vi "PDF_Interface_PDF Protokoll EPA1065_LeakCheck.vi"(8 "error in (no error)":errorcluster caption="Fehler (Eingang, kein Fehler)", 10 "TablePictures Refnum In":refnum<vi>[](array[refnum]), 11 "Save PDF File Path":path) -> (0 "error out":errorcluster caption="Fehler (Ausgang)")   [LabVIEW 2020, in "EPA 1065.lvlib" / "Dichtheitstest 1065-345.lvlib"]
uses:
  Dichtheitstest 1065-345.lvlib
  Versa Button.ctl
  VFS Button.ctl
  Sprachverwaltung/FGV Aktion Tabelle zerlegen.ctl
  Aktion Protokolldaten_Leak check.ctl
  Aktion Leak Daten.ctl
  <vilib>/Utility/miscctls.llb/LVRowAndColumnTypeDef.ctl
  <vilib>/Simplicity AI/SAI_PDF_API/Classes/Context/Controls/SAI_PDF_PDF Details.ctl
  PDF_Interface/PDF Interface Helper/PDFContentType.ctl
  PDF_Interface/PDF Interface Helper/PDFTableContentType.ctl
  PDF_Interface/PDF Interface Helper/PDFResults.ctl
  PDF_Interface/PDF Interface Helper/PDFResultPictures.ctl
  PDF_Interface/PDF Interface Helper/PDFCommentPosition.ctl
  PDF_Interface/PDF Interface Helper/PDFPageBreak.ctl
  PDF_Interface/PDF Interface Helper/PDFTablePictures.ctl
  PDF_Interface/PDF Interface Helper/PDFBemerkung.ctl
  <vilib>/Simplicity AI/SAI_PDF_API/Classes/Context/Controls/SAI_PDF_Text Align.ctl
  <vilib>/Simplicity AI/SAI_PDF_API/Classes/Context/Controls/SAI_PDF_Font.ctl
  <vilib>/Simplicity AI/SAI_PDF_API/Classes/Context/Controls/SAI_PDF_Font Encoding.ctl
  PDF_Interface/PDF Protokoll Standard Kopf Optionen.ctl
  Allgemein/allgemeine Sub-VIs.lvlib
  Sprachverwaltung/Sprachverwaltung.lvlib
  PDF_Interface/PDF Interface.lvlib
  <vilib>/Simplicity AI/SAI_PDF_API/Classes/Context/Context.lvclass
  PDF_Interface/PDF Interface Helper/PDF Interface Helper.lvlib
  Linearisierung V2/Protokoll/Protokoll.lvlib
panel:
  in  "VFS button":T1
  in  "FAS button":T2
  out "EPA Konform":string
  out "Inner diameter \nHL to SP":sgl format="%#_5g"
  out "Length HL to SP":sgl format="%#_5g"
  out "Total volume VFS":sgl
  out "Length HL to VFS":sgl format="%#_5g"
  out "Inner diameter  \nHL to VFS":sgl format="%#_5g"
  out "Total volume versa":sgl caption="Total volume Versa"
  out "Heizleitung\nzum\nVFS":bool caption="Heated line\nto\nVFS"
  out "Heizleitung\nzur\nEntnahmestelle":bool caption="Heated Line\nto\nSampling point"
  out "VFS":bool
  out "Tabelle":string[][](table)
  # "Leak Check - EPA § 1065.345"
  # "mm"
  # "mm"
  # "mm³"
  # "mm"
  # "mm"
  # "mm³"
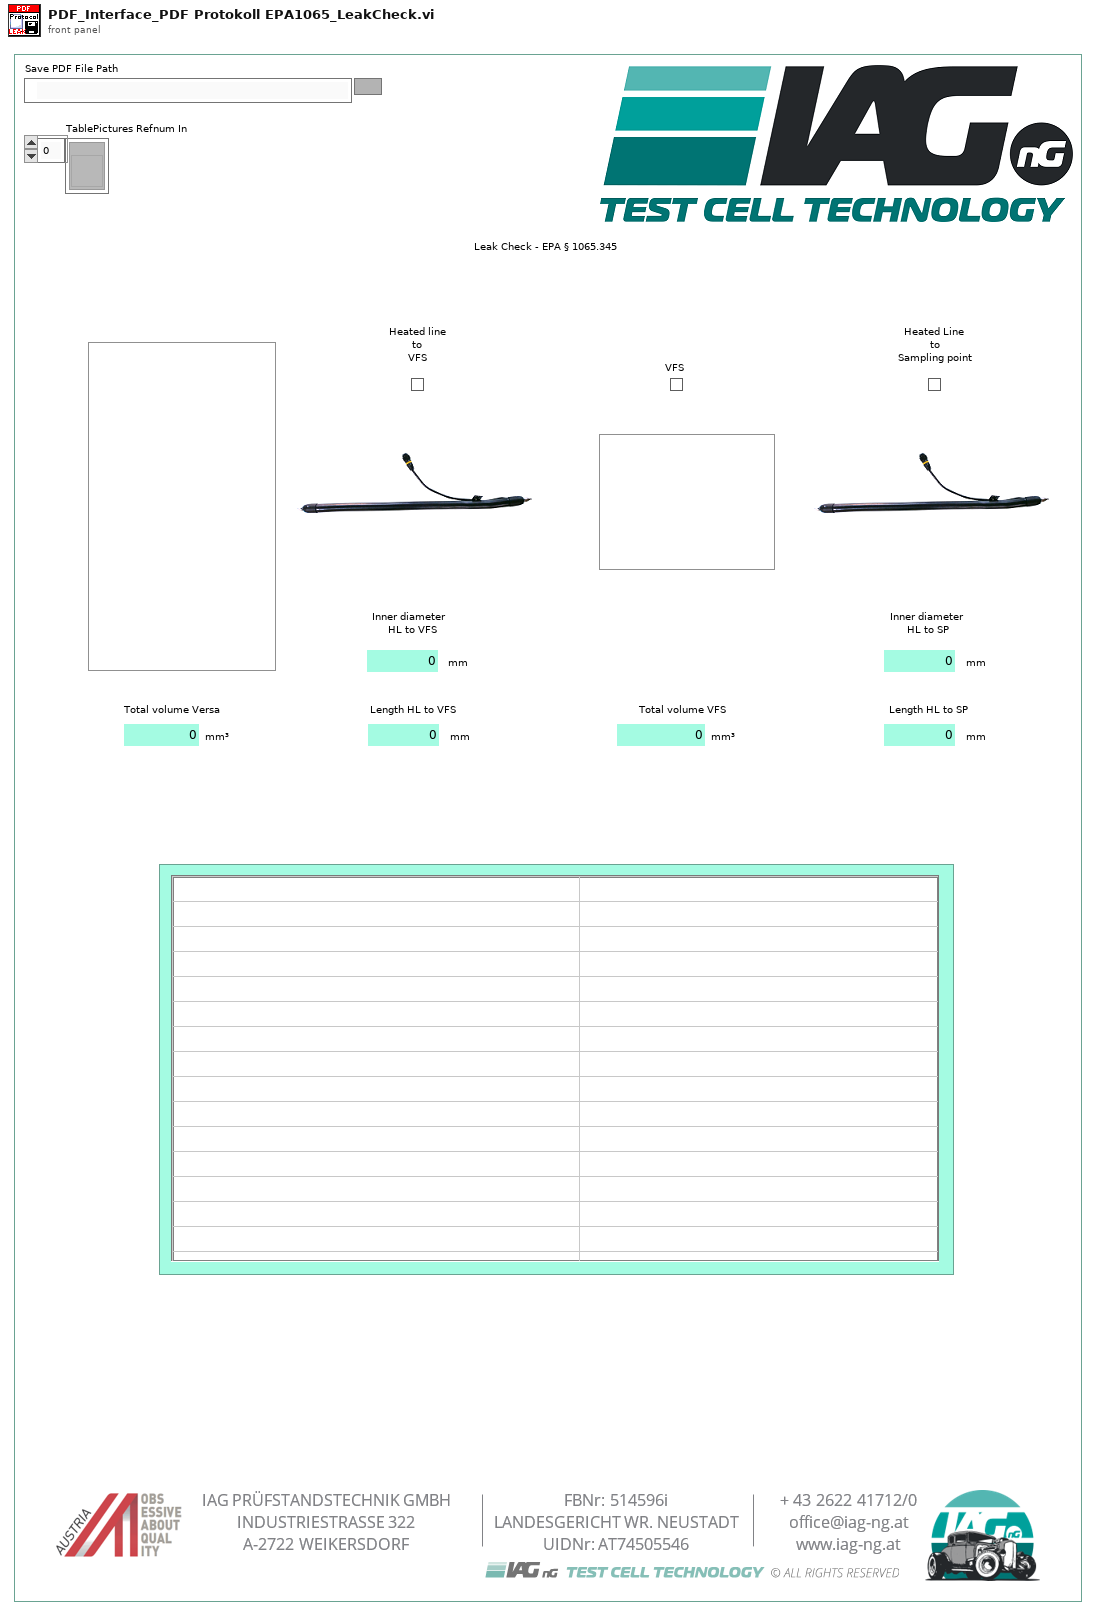
[diagram p1: front panel]
types:
  T1 = typedef "EPA 1065.lvlib/Dichtheitstest 1065-345.lvlib/VFS Button.ctl" = bool
  T2 = typedef "EPA 1065.lvlib/Dichtheitstest 1065-345.lvlib/Versa Button.ctl" = bool
  T3 = typedef "Sprachverwaltung.lvlib/FGV Aktion Tabelle zerlegen.ctl" = enum16{"laden", "vereinzeln", "speichern"}
  T4 = typedef "LVRowAndColumnTypeDef.ctl" = cluster{"Row":i32, "Column":i32}
  T5 = typedef "EPA 1065.lvlib/Dichtheitstest 1065-345.lvlib/Aktion Leak Daten.ctl" = enum16{"lesen", "laden", "speichern", "Volumen", "berechnen", "Leak check aktiv", "Leak Zustand", "Pfad", "Pfad speichern"}
  T6 = typedef "EPA 1065.lvlib/Dichtheitstest 1065-345.lvlib/Aktion Protokolldaten_Leak check.ctl" = enum16{"lesen", "Zeitstempel", "Bearbeiter", "Daten", "Auswertung", "löschen"}
  T7 = typedef "PDF Interface.lvlib/PDF Protokoll Standard Kopf Optionen.ctl" = cluster{"Analysator":bool, "FT-IR Rezept":bool, "Gasteiler":bool, "Gas Komponente":bool, "Gas Flasche":bool, "LIN Protokoll":bool, "Operator":bool}
  T8 = typedef "PDF Interface.lvlib/PDF Interface Helper.lvlib/PDFTablePictures.ctl" = cluster{"Ctl Refnum In":refnum<vi>[], "RowOrColumn":enum16{"Row", "Column"}, "IndexToInsert":u16, "Image Scale (%)":sgl[], "Autoscale? (T)":bool[], "Horizontal Align":i32}
  T9 = typedef "PDF Interface.lvlib/PDF Interface Helper.lvlib/PDFPageBreak.ctl" = enum16{"none", "before", "after", "after comment"}
  T10 = typedef "PDF Interface.lvlib/PDF Interface Helper.lvlib/PDFCommentPosition.ctl" = enum16{"before", "after"}
  T11 = typedef "PDF Interface.lvlib/PDF Interface Helper.lvlib/PDFContentType.ctl" = cluster{"Titel":string, "Header Table":string[][], "Table Array":T12[], "Bemerkungen":T15[]}
  T12 = typedef "PDF Interface.lvlib/PDF Interface Helper.lvlib/PDFTableContentType.ctl" = cluster{"TableHeader":string[], "Table":string[][], "Relative Column Widths (%)":sgl[], "Results":T13, "PositionBemerkung":T10, "PageBreak":T9, "TablePictures":T8, "Horizontal Align":i32}
  T13 = typedef "PDF Interface.lvlib/PDF Interface Helper.lvlib/PDFResults.ctl" = cluster{"Results":cluster{"Result Text":string, "Result":bool}[], "ResultPictures":T14, "use Pictures":bool, "Image Scale (%)":sgl, "Autoscale? (T)":bool, "Horizontal Align":i32, "Position":i32}
  T14 = typedef "PDF Interface.lvlib/PDF Interface Helper.lvlib/PDFResultPictures.ctl" = cluster{"Yes Ctl Refnum":refnum<vi>, "No Ctl Refnum":refnum<vi>}
  T15 = typedef "PDF Interface.lvlib/PDF Interface Helper.lvlib/PDFBemerkung.ctl" = cluster{"Bemerkung Text":string, "Align (Left)":T16, "Add Line Feeds (F:No)":bool, "Font":T17}
  T16 = typedef "SAI_PDF_Toolkit.lvlib/Context.lvclass/SAI_PDF_Text Align.ctl" = i32
  T17 = typedef "SAI_PDF_Toolkit.lvlib/Context.lvclass/SAI_PDF_Font.ctl" = cluster{"Font":string, "Size":i32, "Colour":u32, "Bold":bool, "Italic":bool, "Underline":bool, "Strikethrough":bool, "Font Encoding":T18}
  T18 = typedef "SAI_PDF_Toolkit.lvlib/Context.lvclass/SAI_PDF_Font Encoding.ctl" = enum16{"Cp1252, WinANSI", "IdentityH", "IdentityV", "Cp1250", "Cp1257", "MacRoman"}
  T19 = typedef "SAI_PDF_Toolkit.lvlib/Context.lvclass/SAI_PDF_PDF Details.ctl" = cluster{"Title":string, "Subject":string, "Keywords":string, "Author":string, "Creator":string}
  T20 = cluster{"Header Footer Text Cluster":cluster{"Header Text":string, "Footer Text":string, "Time":string, "Page Number":string}, "PDF Details":T19}
  T21 = typedef "EPA 1065.lvlib/Dichtheitstest 1065-345.lvlib/Gesamtvolumen.ctl" = cluster{"FAS":sgl, "d von HL zu VFS":sgl, "l von HL zu VFS":sgl, "VFS":sgl, "d von HL zu SP":sgl, "l von HL zu SP":sgl, "Heizleitung zum VFS":bool, "VFS a":bool, "Heizleitung zur Entnahmestelle":bool, "Gesamtes Volumen":sgl, "LeakValve":u16, "Einheit":enum16{"mol/s", "mbar"}}
  T22 = typedef "EPA 1065.lvlib/Dichtheitstest 1065-345.lvlib/Leak Protokoll Einstellungen.ctl" = cluster{"Bearbeiter:":string, "Pfad:":path, "Textname:":string, "Analysator":T23}
  T23 = typedef "System Einstellungen V2.lvlib/Analysatoren.ctl" = string
  T24 = cluster{"Header Size":i32, "Column Ratio left":sgl[]}
  T25 = typedef "String - Ausgabefeld.ctl" = string
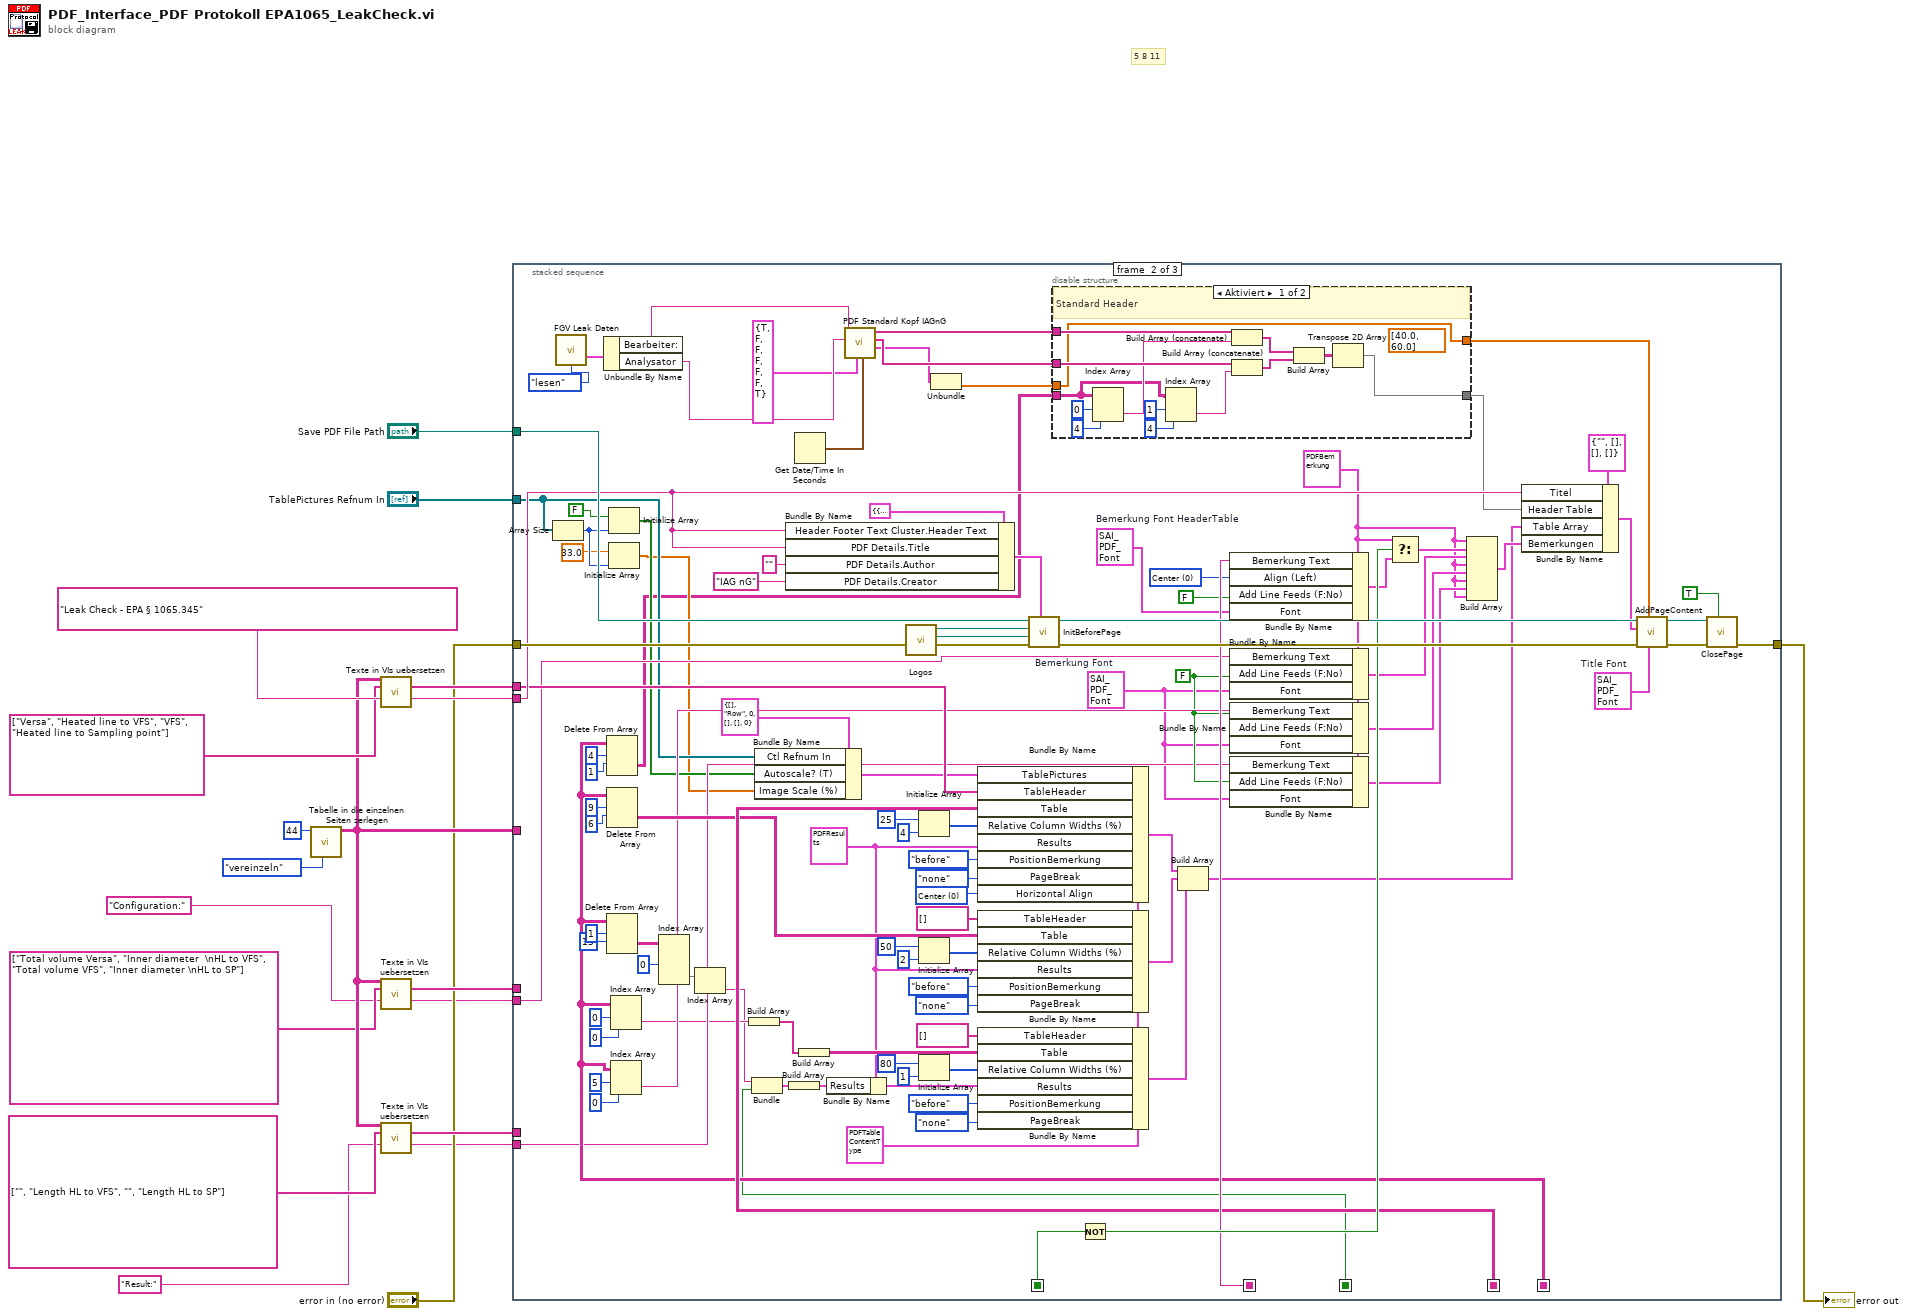
[diagram p0: block diagram]
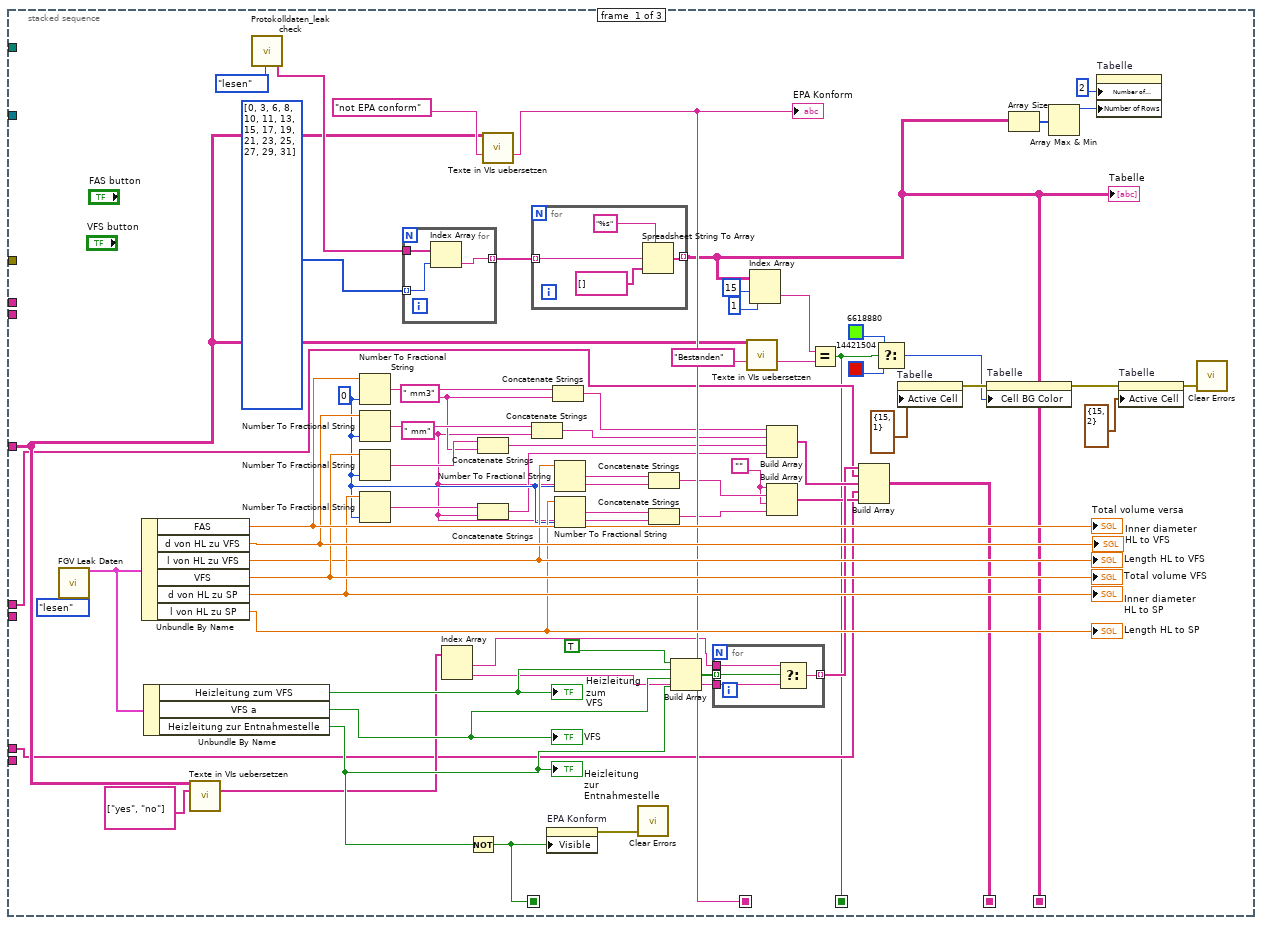
[diagram p2: hidden frame]
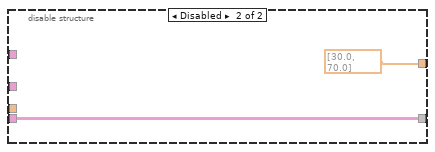
[diagram p3: hidden frame]
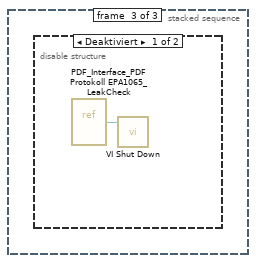
[diagram p4: hidden frame]
diagram:
  # "5 8 11"
  n1 = call "Tabelle in die einzelnen Seiten zerlegen.vi"("Aktion"=FGV_Aktion_Tabelle_zerlegen."vereinzeln", "Index (Seite)"=44) -> ("Sprachliste"=w15:string[][])  [unwired: 7 in, 2 out]
  n2 = call "Texte in VIs uebersetzen.vi"("Sprachliste"=w15, "String-Array zum Übersetzen"=string[] ["Versa", "Heated line to VFS", "VFS", "Heated line to Sampling point"], "String zum Übersetzen"="Leak Check - EPA § 1065.345") -> ("String-Array zum Übersetzen"=w10:string[], "String zum Übersetzen"=w11:string)  [unwired: 8 in, 3 out]
  n3 = call "Texte in VIs uebersetzen.vi"("Sprachliste"=w15, "String-Array zum Übersetzen"=string[] ["Total volume Versa", "Inner diameter  \nHL to VFS", "Total volume VFS", "Inner diameter \nHL to SP"], "String zum Übersetzen"="Configuration:") -> ("String-Array zum Übersetzen"=w12:string[], "String zum Übersetzen"=w4:string)  [unwired: 8 in, 3 out]
  n4 = call "Texte in VIs uebersetzen.vi"("Sprachliste"=w15, "String-Array zum Übersetzen"=string[] ["", "Length HL to VFS", "", "Length HL to SP"], "String zum Übersetzen"="Result:") -> ("String-Array zum Übersetzen"=w9:string[], "String zum Übersetzen"=w2:string)  [unwired: 8 in, 3 out]
  n5 = stacked-sequence {
    seq-local: [w47 _ _] -> [_ w167 _]
    seq-local: [w41 _ _] -> [_ w183 _]
    seq-local: [w40 _ _] -> [_ w145 _]
    seq-local: [w39 _ _] -> [_ w185 _]
    seq-local: [w22 _ _] -> [_ w140 _]
    tunnel: w15 -> [w38 _ _]
    tunnel: w12 -> [w25 _ _]
    tunnel: w11 -> [_ w180 _]
    tunnel: w10 -> [_ w169 _]
    tunnel: w9 -> [w23 _ _]
    tunnel: "Save PDF File Path" -> [_ w189 _]
    tunnel: "error in (no error)" -> [_ w188 _]
    tunnel: [_ w187 _] -> w6
    tunnel: w4 -> [_ w132 _]
    tunnel: w2 -> [_ w129 _]
    tunnel: "TablePictures Refnum In" -> [_ w125 _]
    frame #0 {
      w27 = " mm" ("String")
      w30 = " mm3" ("String")
      w20 = ""
      w48 = i16 0 ("Genauigkeit (6)")
      n6 = call "FGV Leak Daten.vi"("Aktion"=Aktion_Leak_Daten."lesen") -> ("Gesamtvolumen"=w79:T21)  [unwired: 10 in, 4 out]
      n7 = Unbundle By Name(w79) -> ("FAS"=w60:sgl, "d von HL zu VFS"=w58:sgl, "l von HL zu VFS"=w52:sgl, "VFS"=w56:sgl, "d von HL zu SP"=w53:sgl, "l von HL zu SP"=w50:sgl)
      "Total volume versa" <- w60
      "Inner diameter  \nHL to VFS" <- w58
      "Length HL to VFS" <- w52
      "Total volume VFS" <- w56
      "Length HL to SP" <- w50
      "Inner diameter \nHL to SP" <- w53
      n8 = Unbundle By Name(w79) -> ("Heizleitung zum VFS"=w45:bool, "VFS a"=w44:bool, "Heizleitung zur Entnahmestelle"=w43:bool)
      "VFS" <- w44
      "Heizleitung\nzur\nEntnahmestelle" <- w43
      "Heizleitung\nzum\nVFS" <- w45
      n9 = call "Texte in VIs uebersetzen.vi"("Sprachliste"=w38, "String-Array zum Übersetzen"=string[] ["yes", "no"] ("Element")) -> ("String-Array zum Übersetzen"=w36:string[])  [unwired: 9 in, 4 out]
      n10 = call "Protokolldaten_leak check.vi"("Aktion"=Aktion_Protokolldaten_Leak_check."lesen") -> ("Auswertung"=w81:string[])  [unwired: 23 in, 3 out]
      n11 = Number To Fractional String(number=w60, precision (6)=w48) -> (F-format string=w59:string)  [unwired: 2 in]
      n12 = Number To Fractional String(number=w58, precision (6)=w48) -> (F-format string=w57:string)  [unwired: 2 in]
      n13 = Number To Fractional String(number=w56, precision (6)=w48) -> (F-format string=w55:string)  [unwired: 2 in]
      n14 = Number To Fractional String(number=w53, precision (6)=w48) -> (F-format string=w54:string)  [unwired: 2 in]
      n15 = for {
        tunnel: w81 -> [w96]
        tunnel: i32[] [0, 3, 6, 8, 10, 11, 13, 15, 17, 19, 21, 23, 25, 27, 29, 31] -> [w95] mode=indexing
        tunnel: [w94] -> w66 mode=indexing
        n16 = Index Array(array=w96, index=w95) -> (element=w94:string)
      }
      n17 = Index Array(array=w36) -> (element #1=w35:string, element #2=w34:string)  [unwired: 2 in]
      n18 = Not(x=w43) -> (.not. x?=w39:bool)
      n19 = Concatenate Strings(w55, w30) -> (w31:string)
      n20 = Concatenate Strings(w54, w27) -> (w29:string)
      n21 = call "Texte in VIs uebersetzen.vi"("Sprachliste"=w38, "String zum Übersetzen"="not EPA conform" ("EPA Konform")) -> ("String zum Übersetzen"=w41:string)  [unwired: 9 in, 4 out]
      "EPA Konform" <- w41
      n22 = for {
        tunnel: [w92] -> w40 mode=indexing
        tunnel: w66 -> [w90] mode=indexing
        n23 = Spreadsheet String To Array(format string="%s" ("Format-String"), spreadsheet string=w90, array type (2D Dbl)=string[] []) -> (array=w92:string[])  [unwired: 1 in]
      }
      "Tabelle" <- w40
      n24 = Concatenate Strings(w57, w27) -> (w32:string)
      n25 = property on="EPA Konform" class="Str"("Visible"=w39) -> (error out=w63:errorcluster)  [unwired: 2 in, 1 out]
      n26 = Concatenate Strings(w59, w30) -> (w33:string)
      n27 = Number To Fractional String(number=w52, precision (6)=w48) -> (F-format string=w51:string)  [unwired: 2 in]
      n28 = Number To Fractional String(number=w50, precision (6)=w48) -> (F-format string=w49:string)  [unwired: 2 in]
      n29 = call <vilib>:"Clear Errors.vi"("error in (no error)"=w63) -> ()  [unwired: 5 in, 2 out]
      n30 = Concatenate Strings(w51, w27) -> (w28:string)
      n31 = Concatenate Strings(w49, w27) -> (w21:string)
      n32 = Build Array(TRUE, w45, w44, w43) -> (w42:bool[])
      n33 = for {
        tunnel: w42 -> [w89] mode=indexing
        tunnel: [w88] -> w26 mode=indexing
        tunnel: w35 -> [w87]
        tunnel: w34 -> [w86]
        n34 = Select(t=w87, s=w89, f=w86) -> (s? t:f=w88:string)
      }
      n35 = call "Texte in VIs uebersetzen.vi"("Sprachliste"=w38, "String zum Übersetzen"="Bestanden" ("Element")) -> ("String zum Übersetzen"=w76:string)  [unwired: 9 in, 4 out]
      n36 = Index Array(array=w40, index (row)=15 ("Index (Zeile)"), index (col)=1 ("Deaktivierter Index (Spalte)")) -> (element=w74:string)
      n37 = Build Array(w33, w32, w31, w29) -> (w61:string[])
      n38 = Build Array(w20, w28, w20, w21) -> (w24:string[])
      n39 = Equal?(x=w74, y=w76) -> (x = y?=w22:bool)
      n40 = Build Array(w26, w25, w61, w23, w24) -> (w47:string[][])
      n41 = Select(t=u32 6618880, s=w22, f=u32 14421504) -> (s? t:f=w71:u32)
      n42 = property on="Tabelle" class="Tbl (strikt)"("Active Cell"=T4 {"Row"=15, "Column"=1} ("Aktive Zelle:Aktive Zelle")) -> (error out=w72:errorcluster)  [unwired: 2 in, 1 out]
      n43 = property on="Tabelle" class="Tbl (strikt)"(error in=w72, "Cell BG Color"=w71) -> (error out=w70:errorcluster)  [unwired: 1 in, 1 out]
      n44 = Array Size(array=w40) -> (size(s)=w84:i32[])
      n45 = Array Max & Min(array=w84) -> (max value=w83:i32)  [unwired: 3 out]
      n46 = property on="Tabelle" class="Tbl (strikt)"("Number of Columns"=u32 2 ("Spaltenanzahl"), "Number of Rows"=w83) -> ()  [unwired: 2 in, 2 out]
      n47 = property on="Tabelle" class="Tbl (strikt)"(error in=w70, "Active Cell"=T4 {"Row"=15, "Column"=2} ("Aktive Zelle:Aktive Zelle")) -> (error out=w68:errorcluster)  [unwired: 1 in, 1 out]
      n48 = call <vilib>:"Clear Errors.vi"("error in (no error)"=w68) -> ()  [unwired: 5 in, 2 out]
    }
    frame #1 {
      w112 = T15 {"Bemerkung Text"="", "Align (Left)"=0, "Add Line Feeds (F:No)"=FALSE, "Font"={"Font"="Arial", "Size"=10, "Colour"=0, "Bold"=FALSE, "Italic"=FALSE, "Underline"=FALSE, "Strikethrough"=FALSE, "Font Encoding"=enum."Cp1252, WinANSI"}} ("Bemerkung")
      w114 = T13 {"Results"=[], "ResultPictures"={"Yes Ctl Refnum"=refnum, "No Ctl Refnum"=refnum}, "use Pictures"=FALSE, "Image Scale (%)"=100.0, "Autoscale? (T)"=TRUE, "Horizontal Align"=3, "Position"=0} ("Results")
      w116 = T12 {"TableHeader"=[], "Table"=[], "Relative Column Widths (%)"=[], "Results"={"Results"=[], "ResultPictures"={"Yes Ctl Refnum"=refnum, "No Ctl Refnum"=refnum}, "use Pictures"=FALSE, "Image Scale (%)"=0.0, "Autoscale? (T)"=FALSE, "Horizontal Align"=0, "Position"=0}, "PositionBemerkung"=enum."before", "PageBreak"=enum."none", "TablePictures"={"Ctl Refnum In"=[], "RowOrColumn"=enum."Row", "IndexToInsert"=0, "Image Scale (%)"=[], "Autoscale? (T)"=[], "Horizontal Align"=0}, "Horizontal Align"=0} ("Table Array")
      w117 = T16 0 items=["Center", "Justified", "Justified All", "Left", "Right"] ("Align (Left)")
      w130 = FALSE ("Add Line Feeds (F:No)")
      w111 = T17 {"Font"="Arial", "Size"=12, "Colour"=16711680, "Bold"=TRUE, "Italic"=TRUE, "Underline"=FALSE, "Strikethrough"=FALSE, "Font Encoding"=enum."Cp1252, WinANSI"}  # Bemerkung Font HeaderTable
      w110 = T17 {"Font"="Arial", "Size"=12, "Colour"=0, "Bold"=TRUE, "Italic"=TRUE, "Underline"=FALSE, "Strikethrough"=FALSE, "Font Encoding"=enum."Cp1252, WinANSI"}  # Bemerkung Font
      w181 = T17 {"Font"="Arial", "Size"=26, "Colour"=0, "Bold"=TRUE, "Italic"=FALSE, "Underline"=TRUE, "Strikethrough"=FALSE, "Font Encoding"=enum."Cp1252, WinANSI"}  # Title Font
      w182 = T16 0 items=["Center", "Justified", "Justified All", "Left", "Right"] ("Align (Left)")
      n49 = Array Size(array=w125) -> (size(s)=w122:i32)
      n50 = call "FGV Leak Daten.vi"("Aktion"=Aktion_Leak_Daten."lesen") -> ("Leak Protokoll"=w109:T22)  [unwired: 10 in, 4 out]
      n51 = Unbundle By Name(w109) -> ("Bearbeiter:"=w108:string, "Analysator"=w107:T23)
      n52 = Delete From Array(array=w145, length=4 ("Länge"), index (row)=1 ("Index (Zeile)")) -> (deleted portion=w102:string[][])  [unwired: 1 in, 1 out]
      n53 = Delete From Array(array=w145, length=9 ("Länge"), index (row)=6 ("Deaktivierter Index (Spalte)")) -> (deleted portion=w158:string[][])  [unwired: 1 in, 1 out]
      n54 = Delete From Array(array=w145, length=1 ("Länge"), index (row)=15 ("Index (Zeile)")) -> (deleted portion=w144:string[][])  [unwired: 1 in, 1 out]
      n55 = Initialize Array(FALSE, w122) -> (w123:bool[])
      n56 = Initialize Array(sgl 33.0 ("Column Ratio left"), w122) -> (w120:sgl[])
      n57 = Index Array(array=w145, index (row)=0 ("Index (Zeile)"), index (col)=0 ("Deaktivierter Index (Spalte)")) -> (element=w128:string)
      n58 = Index Array(array=w145, index (row)=5 ("Index (Zeile)"), index (col)=0 ("Deaktivierter Index (Spalte)")) -> (element=w133:string)
      n59 = Index Array(array=w144, index (col) #1=0 ("Deaktivierter Index (Spalte)")) -> (element #2=w141:string[])  [unwired: 3 in, 1 out]
      n60 = Index Array(array=w141) -> (element=w127:string)  [unwired: 1 in]
      n61 = Build Array(w128) -> (w126:string[])
      n62 = Bundle("String"=w127, w140) -> (w139:cluster{"String":string, bool})  [unwired: 1 in]
      n63 = Bundle By Name(cluster=T8 {"Ctl Refnum In"=[], "RowOrColumn"=enum."Row", "IndexToInsert"=0, "Image Scale (%)"=[], "Autoscale? (T)"=[], "Horizontal Align"=0} ("TablePictures"), "Ctl Refnum In"=w125, "Autoscale? (T)"=w123, "Image Scale (%)"=w120) -> (w118:T8)
      n64 = Bundle By Name(cluster=T20 {"Header Footer Text Cluster"={"Header Text"="Protokoll XYZ", "Footer Text"="IAG nG", "Time"="<TIMESTAMP yyyy-MM-dd>", "Page Number"="Page <P> of <PT>"}, "PDF Details"={"Title"="Test PDF", "Subject"="Versa Tabasco", "Keywords"="", "Author"="RIW", "Creator"="IAG"}} ("Info"), "Header Footer Text Cluster.Header Text"=w180, "PDF Details.Title"=w180, "PDF Details.Author"="", "PDF Details.Creator"="IAG nG") -> (w192:T20)
      n65 = Build Array(w139) -> (w113:cluster{"String":string, bool}[])
      n66 = Get Date/Time In Seconds() -> (seconds since 1Jan1904=w99:timestamp)
      n67 = Build Array(w126) -> (w142:string[][])
      n68 = Bundle By Name(cluster=w114, "Results"=w113) -> (w115:T13)
      n69 = call "PDF Standard Kopf IAGnG.vi"("Zeitstempel"=w99, "Oprtionen Cluster"=T7 {"Analysator"=TRUE, "FT-IR Rezept"=FALSE, "Gasteiler"=FALSE, "Gas Komponente"=FALSE, "Gas Flasche"=FALSE, "LIN Protokoll"=FALSE, "Operator"=TRUE}, "Analysator"=w107, "Bearbeiter/in"=w108) -> ("Size Cluster"=w98:T24, "Header Values"=w103:T25[], "Header Labels"=w104:string[])  [unwired: 4 in, 1 out]
      n70 = call "Logos.vi"() -> ("Footer Image File Path"=w201:path, "Header Image File Path"=w202:path)  [unwired: 8 in, 2 out]
      n71 = Initialize Array(25, 4 ("Dimensionsgröße")) -> (w177:i32[])
      n72 = Initialize Array(50, 2 ("Dimensionsgröße")) -> (w172:i32[])
      n73 = Initialize Array(80, 1 ("Dimensionsgröße")) -> (w154:i32[])
      n74 = Unbundle(w98) -> ("Column Ratio left"=w97:sgl[])  [unwired: 1 out]
      n75 = Bundle By Name(cluster=w116, "TablePictures"=w118, "TableHeader"=w169, "Table"=w167, "Relative Column Widths (%)"=w177, "Results"=w114, "PositionBemerkung"=PDFCommentPosition."before", "PageBreak"=PDFPageBreak."none", "Horizontal Align"=w117) -> (w166:T12)
      n76 = Bundle By Name(cluster=w116, "TableHeader"=string[] [], "Table"=w158, "Relative Column Widths (%)"=w172, "Results"=w114, "PositionBemerkung"=PDFCommentPosition."before", "PageBreak"=PDFPageBreak."none") -> (w165:T12)
      n77 = Bundle By Name(cluster=w116, "TableHeader"=string[] [], "Table"=w142, "Relative Column Widths (%)"=w154, "Results"=w115, "PositionBemerkung"=PDFCommentPosition."before", "PageBreak"=PDFPageBreak."none") -> (w138:T12)
      n78 = call "InitBeforePage.vi"("Info"=w192, "Fehler (Eingang, kein Fehler)"=w188, "Footer Image File Path"=w201, "Header Image File Path"=w202, "Path (Dialog if Empty)"=w189) -> ("Fehler (Ausgang)"=w200:errorcluster, "Context (Ausgang)"=w199:refnum<class "Context.lvclass">)  [unwired: 5 in]
      n79 = disable-structure shown="Aktiviert" {
        disable-tunnel: w104 -> [w216 _]
        disable-tunnel: w103 -> [w215 _]
        disable-tunnel: w102 -> [w211 w218]
        disable-tunnel: [w204 w218] -> w101
        disable-tunnel: [w203 sgl[] [30.0, 70.0] ("Column Ratio left")] -> w100
        disable-tunnel: w97 -> [w203 _]
        frame Enabled {
          (unwired) sgl[] [40.0, 60.0] ("Column Ratio left")
          # "Standard Header"
          n80 = Index Array(array=w211, index (row)=0 ("Index (Zeile)"), index (col)=4 ("Deaktivierter Index (Spalte)")) -> (element=w212:string)
          n81 = Index Array(array=w211, index (row)=1 ("Index (Zeile)"), index (col)=4 ("Deaktivierter Index (Spalte)")) -> (element=w208:string)
          n82 = Build Array (concatenate)(w216, w212) -> (w207:string[])
          n83 = Build Array (concatenate)(w215, w208) -> (w206:T25[])
          n84 = Build Array(w207, w206) -> (w205:T25[][])
          n85 = Transpose 2D Array(2D array=w205) -> (transposed array=w204:T25[][])
        }
        frame Disabled {
        }
      }
      n86 = Not(x=w185) -> (.not. x?=w184:bool)
      n87 = Build Array(w166, w165, w138) -> (w164:T12[])
      n88 = Bundle By Name(cluster=w112, "Bemerkung Text"=w183, "Align (Left)"=w182, "Add Line Feeds (F:No)"=FALSE, "Font"=w111) -> (w137:T15)
      n89 = Bundle By Name(cluster=w112, "Bemerkung Text"=w132, "Add Line Feeds (F:No)"=w130, "Font"=w110) -> (w136:T15)
      n90 = Bundle By Name(cluster=w112, "Bemerkung Text"=w133, "Add Line Feeds (F:No)"=w130, "Font"=w110) -> (w135:T15)
      n91 = Bundle By Name(cluster=w112, "Bemerkung Text"=w129, "Add Line Feeds (F:No)"=w130, "Font"=w110) -> (w134:T15)
      n92 = Select(t=w112, s=w184, f=w137) -> (s? t:f=w163:T15)
      n93 = Build Array(w112, w163, w136, w112, w135, w112, w134, w112) -> (w186:T15[])
      n94 = Bundle By Name(cluster=T11 {"Titel"="", "Header Table"=[], "Table Array"=[], "Bemerkungen"=[]} ("Content"), "Titel"=w180, "Header Table"=w101, "Table Array"=w164, "Bemerkungen"=w186) -> (w190:T11)
      n95 = call "AddPageContent.vi"("Title Font"=w181, "Column Ratio left"=w100, "error in"=w200, "Content"=w190, "Context (Eingang)"=w199) -> ("error out"=w198:errorcluster, "Context (Ausgang)"=w197:refnum<class "Context.lvclass">)  [unwired: 5 in]
      n96 = call "ClosePage.vi"("popup viewer"=TRUE, "Fehler (Eingang, kein Fehler)"=w198, "Context (Eingang)"=w197) -> ("Fehler (Ausgang)"=w187:errorcluster)  [unwired: 8 in]
    }
    frame #2 {
      n97 = disable-structure shown="Deaktiviert" {
        frame Disabled {
          n98 = vi-ref "PDF_Interface_PDF Protokoll EPA1065_LeakCheck.vi"() -> (w219:refnum<vi>)
          n99 = call "VI Shut Down.vi"("VI Referenz"=w219) -> ()  [unwired: 11 in]
        }
        frame Enabled {
        }
      }
    }
  }
  "error out" <- w6
